vi "UPS低电量告警参数配置.vi"(11 "监测项描述":string) -> ()   [LabVIEW 2016, in "环境动力监测库.lvlib" / "UPS库.lvlib"]
panel:
  in  "功能启用":bool caption="低电量报警启用"
  in  "UPS电量告警":dbl caption="%"
  # "UPS参数配置"
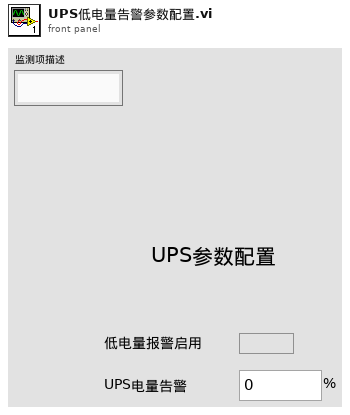
[diagram p1: front panel]
types:
  T1 = cluster{"VISA resource name":refnum<visa-resource-name>, "Serial Config":cluster{"baud rate (9600)":u32, "stop bits (10: 1 bit)":u16, "parity (0:none)":enum16{"None", "Odd", "Even", "Mark", "Space"}, "data bits (8)":u16, "timeout (10sec)":u32}, "型号选择":enum16{"山特UPSC1~3", "山特UPSC6~20", "华为UPS2000-G-(1-3KVA)"}, "HW-UPS-2000 MB session":refnum<class "MB_Master.lvclass">, "连接方式":enum16{"串口", "TCP"}, "IP":string, "Port":string, "低电量报警阈值":u16, "功能启用":bool}
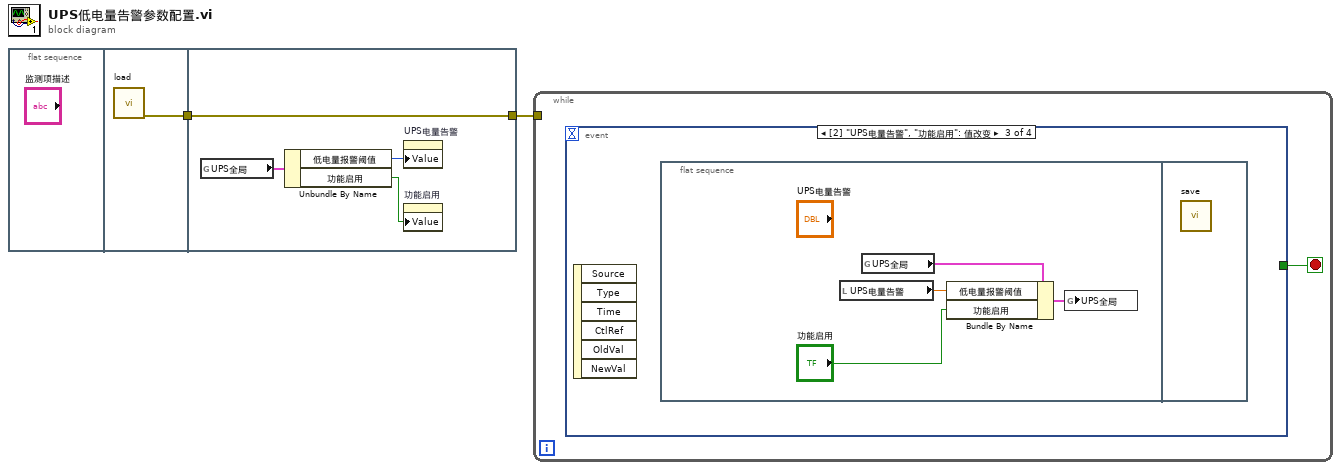
[diagram p0: block diagram]
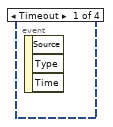
[diagram p2: hidden frame]
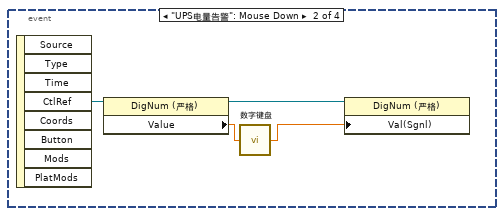
[diagram p3: hidden frame]
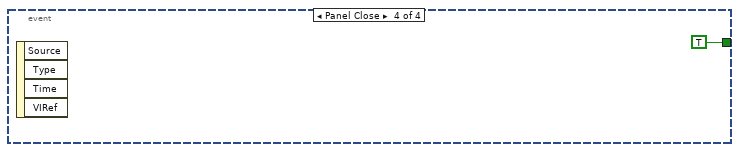
[diagram p4: hidden frame]
diagram:
  n1 = flat-sequence {
    tunnel: [w3] -> w2
    tunnel: [w7] -> w1
    tunnel: w2 -> [w7]
    frame #0 {
    }
    frame #1 {
      n2 = call "load.vi"() -> ("error out"=w3:errorcluster)  [unwired: 11 in]
    }
    frame #2 {
      n3 = global read "断电保存全局变量.vi" "UPS全局"() -> (w6:T1)
      n4 = Unbundle By Name(w6) -> ("低电量报警阈值"=w5:u16, "功能启用"=w4:bool)
      n5 = property on="UPS电量告警" class="DigNum (严格)"("Value"=w5) -> ()  [unwired: 2 in, 2 out]
      n6 = property on="功能启用" class="Bool (严格)"("Value"=w4) -> ()  [unwired: 2 in, 2 out]
    }
  }
  n7 = while {
    tunnel: w1 -> [_]
    stop <- w8 stop-if-true
    n8 = event shown="[2] \"UPS电量告警\", \"功能启用\": 值改变" {
      selector: _ -> [_ _ _ _]
      dyn-events: _ -> [_ _ _ _]
      timeout: _ -> [_ _ _ _]
      tunnel: [_ _ _ TRUE] -> w8
      event Timeout {
        n9 = event-data() -> ()  [unwired: 1 in, 3 out]
      }
      event "UPS电量告警": Mouse Down {
        n10 = event-data() -> ("CtlRef"=w9:refnum<vi>)  [unwired: 1 in, 7 out]
        n11 = property class="DigNum (严格)"(reference=w9) -> (reference out=w11:refnum<vi>, "Value"=w12:dbl)  [unwired: 1 in, 1 out]
        n12 = call "数字键盘.vi"("OldNumber"=w12) -> ("NewNumber"=w10:sgl)
        n13 = property class="DigNum (严格)"(reference=w11, "Val(Sgnl)"=w10) -> ()  [unwired: 1 in, 2 out]
      }
      event "UPS电量告警", "功能启用": Value Change {
        n14 = event-data() -> ()  [unwired: 1 in, 6 out]
        n15 = flat-sequence {
          frame #0 {
            n16 = local read "UPS电量告警"() -> (w15:dbl)
            n17 = global read "断电保存全局变量.vi" "UPS全局"() -> (w16:T1)
            n18 = Bundle By Name(cluster=w16, "低电量报警阈值"=w15, "功能启用"="功能启用") -> (w14:T1)
            n19 = global write "断电保存全局变量.vi" "UPS全局"(w14) -> ()
          }
          frame #1 {
            n20 = call "save.vi"() -> ()  [unwired: 11 in, 1 out]
          }
        }
      }
      event Panel Close {
        n21 = event-data() -> ()  [unwired: 1 in, 4 out]
      }
    }
  }
